vi "PipBoy_InitUserEvents.vi"(8 "error in (no error)":errorcluster) -> (0 "error out":errorcluster, 1 "UE-UpdateData":refnum<event-registration>, 2 "UE-PipBoyCmd":refnum<event-registration>, 3 "UE-UpdateData":refnum<user-event>, 5 "UE-PipboyCommand":refnum<user-event>)   [LabVIEW 2014]
uses:
  ctls/PipBoy_PipBoyCommand.ctl
  ctls/PipBoy_Message.ctl
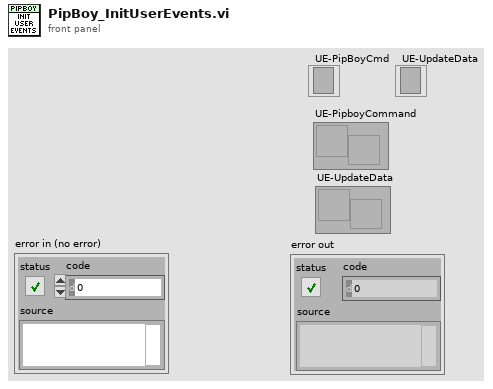
[diagram p1: front panel]
types:
  T1 = typedef "PipBoy_Message.ctl" = cluster{"Name":string, "Data":variant}
  T2 = typedef "PipBoy_PipBoyCommand.ctl" = cluster{"Name":string}
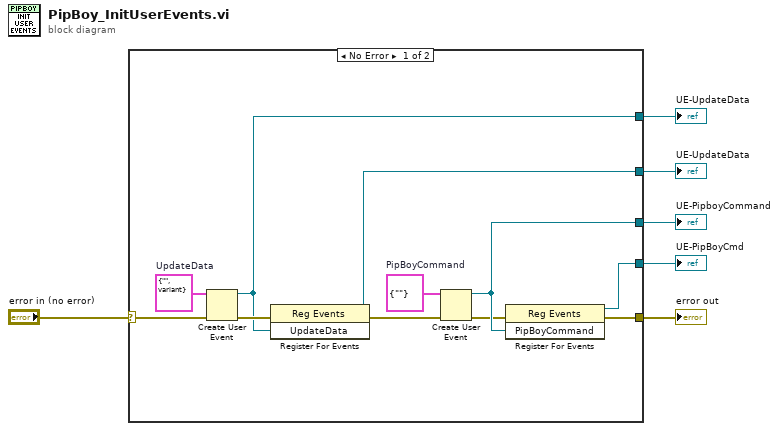
[diagram p0: block diagram]
diagram:
  n1 = case shown="No Error" "error in (no error)" {
    selector: "error in (no error)" -> [w14 w18]
    tunnel: [w16 w18] -> w5
    tunnel: [w15 _] -> w4
    tunnel: [w8 _] -> w3
    tunnel: [w11 _] -> w2
    tunnel: [w7 _] -> w1
    frame No Error {
      w12 = T1 {"Name"="", "Data"=variant}  # UpdateData
      w17 = T2 {"Name"=""}  # PipBoyCommand
      n2 = Create User Event(user event datatype=w12, error in=w14) -> (user event=w8:refnum<user-event>, error out=w10:errorcluster)
      n3 = register-events(error in=w10, w8) -> (reference out=w7:refnum<event-registration>, error out=w9:errorcluster)  [unwired: 1 in]
      n4 = Create User Event(user event datatype=w17, error in=w9) -> (user event=w15:refnum<user-event>, error out=w13:errorcluster)
      n5 = register-events(error in=w13, w15) -> (reference out=w11:refnum<event-registration>, error out=w16:errorcluster)  [unwired: 1 in]
    }
    frame Error {
    }
  }
  "error out" <- w5
  "UE-PipboyCommand" <- w4
  "UE-UpdateData" <- w3
  "UE-PipBoyCmd" <- w2
  "UE-UpdateData" <- w1
